vi "Get Variables.vi"(8 "error in (no error)":errorcluster, 11 "Booelan Operations in":refnum<class "Boolean Functions.lvclass">) -> (0 "error out":errorcluster, 2 "Variables":variant, 3 "Booelan Operations out":refnum<class "Boolean Functions.lvclass">)   [LabVIEW 2019, in "Boolean Functions.lvclass"]
uses:
  Boolean Functions.lvclass
  Boolean Functions.lvclass/Boolean Functions.ctl
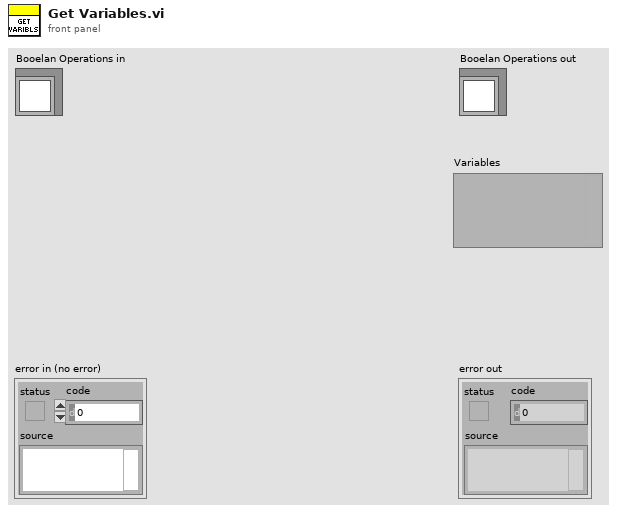
[diagram p1: front panel]
types:
  T1 = typedef "Boolean Operations.lvclass/Variables.ctl" = cluster{"Var1":bool, "Var2":bool}
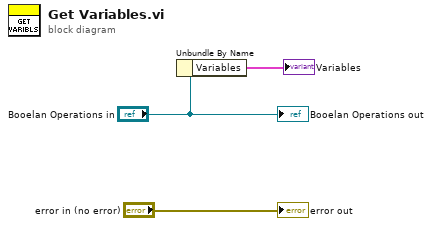
[diagram p0: block diagram]
diagram:
  n1 = Unbundle By Name("Booelan Operations in") -> ("Variables"=→"Variables":T1)
  "error out" <- "error in (no error)"
  "Booelan Operations out" <- "Booelan Operations in"
